vi "PidLowFirstHmi.vi"() -> ()   [LabVIEW 2018, in "Pid.lvlib"]
uses:
  Pid.lvlib
  <vilib>/Platform/TimedLoop/XDataNode/timing_clust.ctl
  <vilib>/Platform/TimedLoop/XDataNode/nitl_modes.ctl
  <vilib>/Platform/TimedLoop/XDataNode/wakeup.ctl
  <vilib>/platform/TimedLoop/XDataNode/XDataNode.xnode
  <vilib>/Platform/TimedLoop/XDataNode/XDNodeRunTimeDep.lvlib
panel:
  in  "Tune with T":bool
  in  "Update now":bool
  in  "Update rate":dbl(slide) scale=0.0..10.0
  out "Loop and out":errorcluster
  out "Modbus":errorcluster
  out "File":errorcluster
  in  "Scale":bool
  in  "Apply Max time":bool
  in  "Max time":dbl
  in  "Start/stop file":bool
  in  "Td":bool
  in  "Ti":bool
  in  "Kd":bool
  in  "Ki":bool
  in  "Kp":bool
  in  "Set Td":sgl
  in  "Set Ti":sgl
  in  "Set Ki":sgl
  in  "Set Kp":sgl
  in  "Set Kd":sgl
  out "Current Td":sgl
  out "Current Ti":sgl
  out "Current Kd":sgl
  out "Current Ki":sgl
  out "Current Kp":sgl
  out "Single Update (Multiple Plots, stacked)":cluster{"Temperature":sgl, "Setpoint":sgl, sgl}(graph)
  out "Time (ms)":u32
  out "Logging to file":bool
  in  "disable buffering (F)":bool
  out "Canceled":bool
  in  "Delimiter":string(combo)
  in  "Format":string(combo)
  out "Communication Failure":bool
  out "Off Hook":bool
  out "Updating":bool
  in  "Frequency":dbl(slide) scale=1.0..100.0
  in  "Stop":bool
  out "Counter":i32
  out "Interval":i64
  in  "file path (use dialog)":path
  in  "Setpoint":bool
  in  "Setpoint":sgl(slide) scale=0.0..255.0
  in  "Manual":bool
  in  "Manual":i16(slide) scale=0.0..255.0
  out "Setpoint":sgl(knob) scale=0.0..300.0
  out "Manual":i16(knob) scale=0.0..255.0
  out "Output":i16(knob) scale=0.0..255.0
  out "Temperature":sgl(slide) scale=0.0..300.0
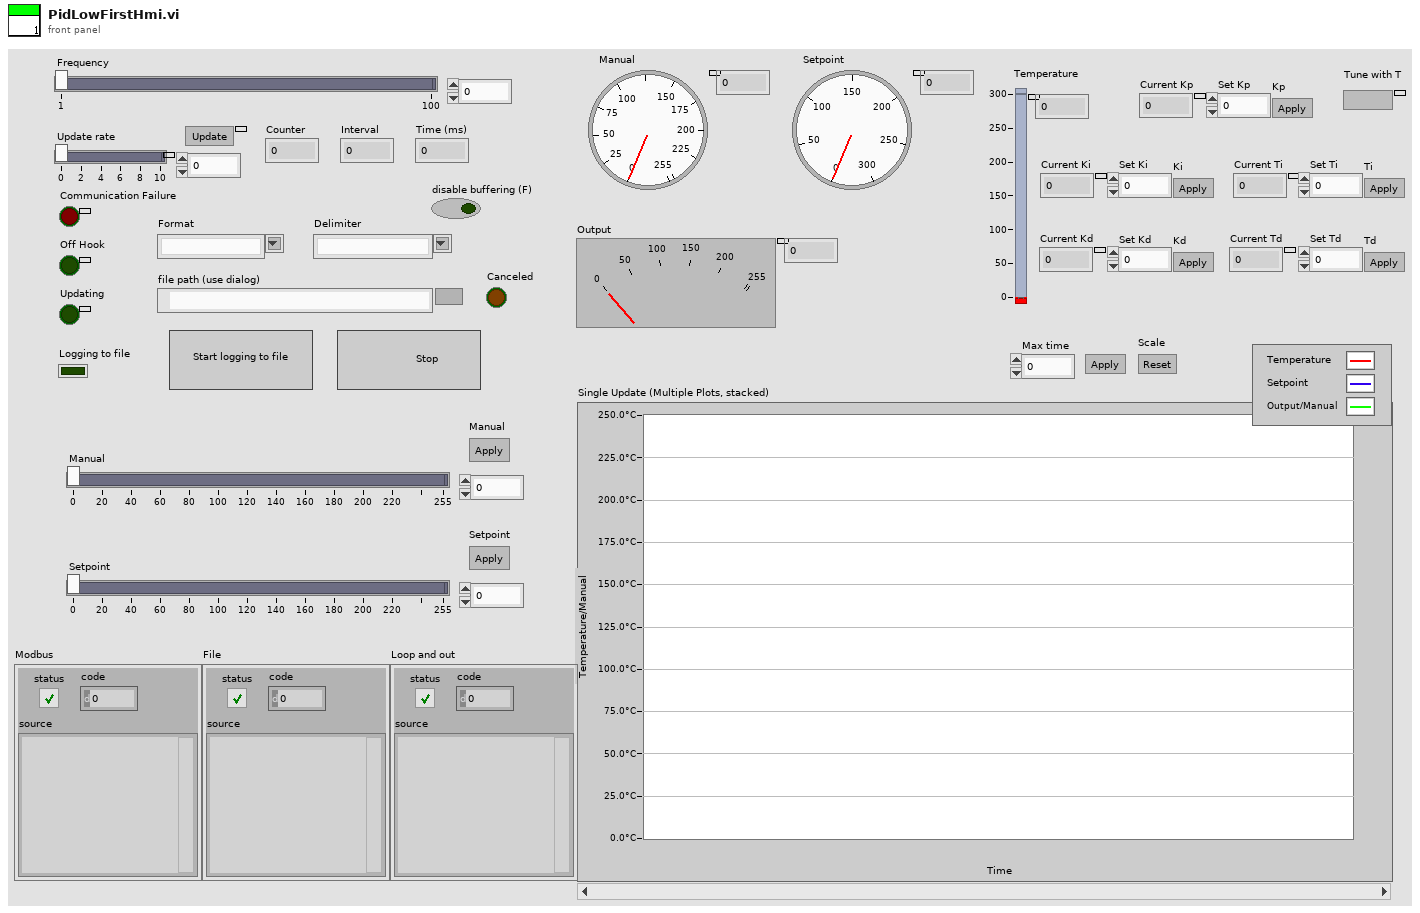
[diagram p1: front panel]
types:
  T1 = enum16{"open", "replace", "create", "open or create", "replace or create", "replace or create with confirmation"}
  T2 = typedef "XDNodeRunTimeDep.lvlib/timing_clust.ctl" = cluster{"Expected End [f-1]":u64, "Actual End [f-1]":u64, "Finished Late? [f-1]":bool, "Expected End [i-1]":u64, "Actual End [i-1]":u64, "Finished Late? [i-1]":bool, "Expected Start [i]":u64, "Actual Start [i]":u64, "Expected Start [f]":u64, "Actual Start [f]":u64, "Source Name":string, "Structure Name":string, "Period":i64, "Deadline":i64, "Offset":i64, "Start":i64, "Priority":i32, "Timeout":i32, "Mode":T3, "Wakeup Reason":T4, "Error":errorcluster, "Source Type":string, "Secondary Source Type":string, "Global End Time":u64, "Global Start Time":u64, "Frame Duration":u64, "Iteration Duration":u64, "Assigned CPU":i32, "I/O Scan Engine Mode":u32}
  T3 = typedef "XDNodeRunTimeDep.lvlib/nitl_modes.ctl" = enum32{"No Change", "Process missed periods, maintain original phase", "Discard missed periods, maintain original phase", "Process missed periods, ignore original phase", "Discard missed periods, ignore original phase"}
  T4 = typedef "XDNodeRunTimeDep.lvlib/wakeup.ctl" = enum32{"Normal", "Aborted", "Asynchronous wakeup", "Timing source error", "Timed loop error", "Timeout"}
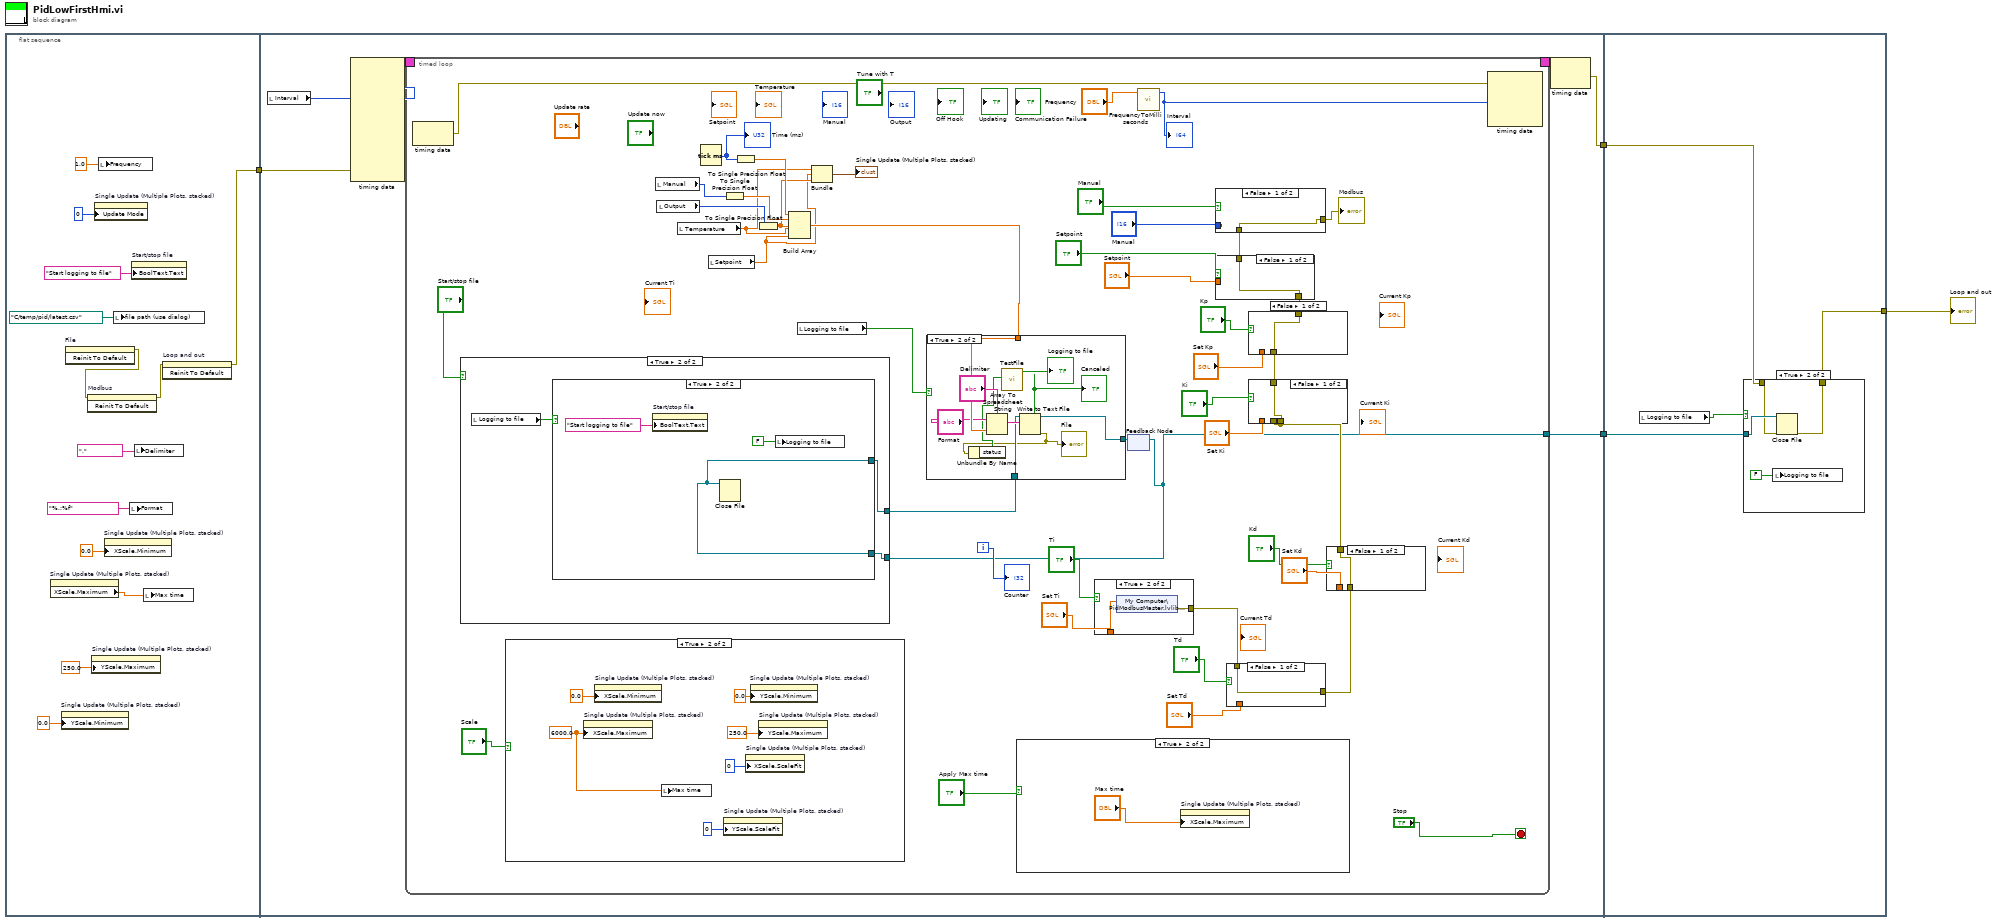
[diagram p0: block diagram]
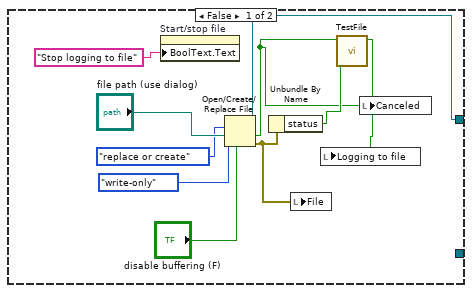
[diagram p5: hidden frame]
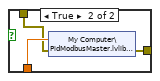
[diagram p6: hidden frame]
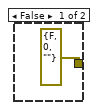
[diagram p7: hidden frame]
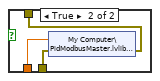
[diagram p8: hidden frame]
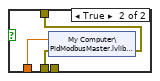
[diagram p9: hidden frame]
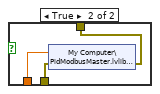
[diagram p10: hidden frame]
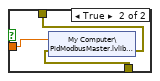
[diagram p11: hidden frame]
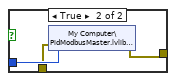
[diagram p13: hidden frame]
diagram:
  n1 = flat-sequence {
    tunnel: [w7] -> w1
    tunnel: [w20] -> w4
    tunnel: [w19] -> w3
    tunnel: w1 -> [w18]
    tunnel: w4 -> [w142]
    tunnel: w3 -> [w143]
    tunnel: [w141] -> w2
    frame #0 {
      n2 = property on="Single Update (Multiple Plots, stacked)" class="WFChart (strict)"() -> ("XScale.Maximum"=w13:dbl)  [unwired: 2 in, 2 out]
      n3 = property on="Single Update (Multiple Plots, stacked)" class="WFChart (strict)"("YScale.Minimum"=0.0 ("Y Scale.Range:Minimum")) -> ()  [unwired: 2 in, 2 out]
      n4 = invoke on="File" class="Clust (strict)" method="Reinit To Default"() -> (error out=w9:errorcluster)  [unwired: 3 in, 2 out]
      n5 = invoke on="Modbus" class="Clust (strict)" method="Reinit To Default"(error in=w9) -> (error out=w8:errorcluster)  [unwired: 2 in, 2 out]
      n6 = property on="Single Update (Multiple Plots, stacked)" class="WFChart (strict)"("YScale.Maximum"=250.0 ("Y Scale.Range:Maximum")) -> ()  [unwired: 2 in, 2 out]
      n7 = property on="Single Update (Multiple Plots, stacked)" class="WFChart (strict)"("Update Mode"=u8 0) -> ()  [unwired: 2 in, 2 out]
      n8 = local write "Frequency"(1.0 ("Frequency")) -> ()
      n9 = property on="Single Update (Multiple Plots, stacked)" class="WFChart (strict)"("XScale.Minimum"=0.0 ("X Scale.Range:Minimum")) -> ()  [unwired: 2 in, 2 out]
      n10 = local write "file path (use dialog)"(path "C:/temp/pid/latest.csv" ("file path (use dialog)")) -> ()
      n11 = local write "Format"("%.;%f" ("Format")) -> ()
      n12 = property on="Start/stop file" class="Bool"("BoolText.Text"="Start logging to file" ("Boolean Text.Text")) -> ()  [unwired: 2 in, 2 out]
      n13 = local write "Delimiter"("," ("Delimiter")) -> ()
      n14 = local write "Max time"(w13) -> ()
      n15 = invoke on="Loop and out" class="Clust (strict)" method="Reinit To Default"(error in=w8) -> (error out=w7:errorcluster)  [unwired: 2 in, 2 out]
    }
    frame #1 {
      n16 = local read "Interval"() -> (w21:i64)
      n17 = node-c288(w21, w18) -> (w23:T2)  [unwired: 8 in]
      n18 = timed-loop {
        timing: w23 -> [_]
        timing-out: [_] -> w22
        tunnel: [w35] -> w19
        i -> [w64]
        stop <- "Stop" stop-if-true
        n19 = node-c288() -> (w26:errorcluster)  [unwired: 1 in]
        n20 = case shown="True" "Scale" {
          frame False {
          }
          frame True {
            w70 = 6000.0 ("X Scale.Range:Maximum")
            n21 = property on="Single Update (Multiple Plots, stacked)" class="WFChart (strict)"("XScale.Maximum"=w70) -> ()  [unwired: 2 in, 2 out]
            n22 = property on="Single Update (Multiple Plots, stacked)" class="WFChart (strict)"("XScale.Minimum"=0.0 ("X Scale.Range:Minimum")) -> ()  [unwired: 2 in, 2 out]
            n23 = local write "Max time"(w70) -> ()
            n24 = property on="Single Update (Multiple Plots, stacked)" class="WFChart (strict)"("YScale.ScaleFit"=u8 0 ("Y Scale.Scale Fit")) -> ()  [unwired: 2 in, 2 out]
            n25 = property on="Single Update (Multiple Plots, stacked)" class="WFChart (strict)"("XScale.ScaleFit"=u8 0 ("X Scale.Scale Fit")) -> ()  [unwired: 2 in, 2 out]
            n26 = property on="Single Update (Multiple Plots, stacked)" class="WFChart (strict)"("YScale.Minimum"=0.0 ("Y Scale.Range:Minimum")) -> ()  [unwired: 2 in, 2 out]
            n27 = property on="Single Update (Multiple Plots, stacked)" class="WFChart (strict)"("YScale.Maximum"=250.0 ("Y Scale.Range:Maximum")) -> ()  [unwired: 2 in, 2 out]
          }
        }
        n28 = local read "Manual"() -> (w39:i16)
        n29 = local read "Output"() -> (w40:i16)
        n30 = local read "Temperature"() -> (w33:sgl)
        n31 = Tick Count (ms)() -> (millisecond timer value=w59:u32)
        "Time (ms)" <- w59
        n32 = local read "Setpoint"() -> (w31:sgl)
        n33 = To Single Precision Float(number=w39) -> (single precision float=w58:sgl)
        n34 = To Single Precision Float(number=w59) -> (single precision float=w60:sgl)
        n35 = To Single Precision Float(number=w40) -> (single precision float=w32:sgl)
        n36 = Build Array(w60, w58, w32, w33, w31) -> (w61:sgl[])
        n37 = local read "Logging to file"() -> (w34:bool)
        n38 = Bundle("Temperature"=w33, "Setpoint"=w31, w32) -> (→"Single Update (Multiple Plots, stacked)":cluster{"Temperature":sgl, "Setpoint":sgl, sgl})  [unwired: 1 in]
        n39 = case shown="True" "Apply Max time" {
          frame False {
          }
          frame True {
            n40 = property on="Single Update (Multiple Plots, stacked)" class="WFChart (strict)"("XScale.Maximum"="Max time") -> ()  [unwired: 2 in, 2 out]
          }
        }
        n41 = case shown="True" "Ti" {
          tunnel: "Set Ti" -> [_ w97]
          tunnel: [errorcluster {"status"=FALSE, "code"=0, "source"=""} ("error IO") w96] -> w25
          frame False {
          }
          frame True {
            n42 = shared-variable "My Computer\\PidModbusMaster.lvlib\\F400010"(w97) -> (error out=w96:errorcluster)  [unwired: 1 in]
          }
        }
        n43 = feedback #1() -> (w35:refnum<file>)  [unwired: 1 in]
        n44 = case shown="True" "Start/stop file" {
          tunnel: [w74 w76] -> w38
          tunnel: w35 -> [w74 w75]
          frame False {
          }
          frame True {
            n45 = local read "Logging to file"() -> (w77:bool)
            n46 = case shown="True" w77 {
              tunnel: [w81 w89] -> w76
              tunnel: w75 -> [_ w89]
              frame False {
                n47 = property on="Start/stop file" class="Bool"("BoolText.Text"="Stop logging to file" ("Boolean Text.Text")) -> ()  [unwired: 2 in, 2 out]
                n48 = Open/Create/Replace File(file path (use dialog)="file path (use dialog)", operation (0:open)=T1."replace or create", access (0:read/write)=enum16{"read/write", "read-only", "write-only"}."write-only", disable buffering (F)="disable buffering (F)") -> (refnum out=w81:refnum<file>, cancelled=w82:bool, error out=w78:errorcluster)  [unwired: 2 in]
                n49 = Unbundle By Name(w78) -> ("status"=w83:bool)
                n50 = local write "File"(w78) -> ()
                n51 = call "TestFile.vi"("status"=w83, "cancelled"=w82) -> ("IsOpen"=w84:bool)  [unwired: 9 in]
                n52 = local write "Logging to file"(w84) -> ()
                n53 = local write "Canceled"(w82) -> ()
              }
              frame True {
                n54 = property on="Start/stop file" class="Bool"("BoolText.Text"="Start logging to file" ("Boolean Text.Text")) -> ()  [unwired: 2 in, 2 out]
                n55 = Close File(refnum=w89) -> ()  [unwired: 1 in, 2 out]
                n56 = local write "Logging to file"(FALSE ("Logging to file")) -> ()
              }
            }
          }
        }
        n57 = case shown="True" w34 {
          tunnel: w61 -> [_ w124]
          tunnel: [w114 w121] -> w36
          tunnel: w38 -> [w114 w119]
          frame False {
          }
          frame True {
            n58 = Array To Spreadsheet String(delimiter (Tab)="Delimiter", array=w124, 3:"Format") -> (spreadsheet string=w120:string)
            n59 = Write to Text File(file (use dialog)=w119, text=w120) -> (refnum out=w121:refnum<file>, cancelled=w117:bool, error out=w115:errorcluster)  [unwired: 2 in]
            "Canceled" <- w117
            "File" <- w115
            n60 = Unbundle By Name(w115) -> ("status"=w116:bool)
            n61 = call "TestFile.vi"("status"=w116, "cancelled"=w117) -> ("IsOpen"=→"Logging to file":bool)  [unwired: 9 in]
          }
        }
        n62 = feedback-in #1(w36) -> ()
        n63 = call "FrequencyToMilliseconds.vi"("Frequency"="Frequency") -> ("Numeric"=w65:i64)  [unwired: 10 in]
        "Interval" <- w65
        n64 = case shown="False" "Td" {
          tunnel: "Set Td" -> [_ w94]
          tunnel: [w91 w93] -> w45
          tunnel: w25 -> [w91 w92]
          frame False {
          }
          frame True {
            n65 = shared-variable "My Computer\\PidModbusMaster.lvlib\\F400012"(w94, error in=w92) -> (error out=w93:errorcluster)
          }
        }
        n66 = case shown="False" "Kd" {
          tunnel: "Set Kd" -> [_ w101]
          tunnel: w45 -> [w98 w100]
          tunnel: [w98 w99] -> w41
          frame False {
          }
          frame True {
            n67 = shared-variable "My Computer\\PidModbusMaster.lvlib\\F400008"(w101, error in=w100) -> (error out=w99:errorcluster)
          }
        }
        n68 = case shown="False" "Ki" {
          tunnel: "Set Ki" -> [_ w105]
          tunnel: w41 -> [_ w104]
          tunnel: [w102 w103] -> w44
          tunnel: w41 -> [w102 _]
          frame False {
          }
          frame True {
            n69 = shared-variable "My Computer\\PidModbusMaster.lvlib\\F400006"(w105, error in=w104) -> (error out=w103:errorcluster)
          }
        }
        n70 = case shown="False" "Kp" {
          tunnel: "Set Kp" -> [_ w109]
          tunnel: w44 -> [w106 w108]
          tunnel: [w106 w107] -> w43
          frame False {
          }
          frame True {
            n71 = shared-variable "My Computer\\PidModbusMaster.lvlib\\F400004"(w109, error in=w108) -> (error out=w107:errorcluster)
          }
        }
        n72 = case shown="False" "Setpoint" {
          tunnel: "Setpoint" -> [_ w113]
          tunnel: w43 -> [w110 w112]
          tunnel: [w110 w111] -> w42
          frame False {
          }
          frame True {
            n73 = shared-variable "My Computer\\PidModbusMaster.lvlib\\F400002"(w113, error in=w112) -> (error out=w111:errorcluster)
          }
        }
        n74 = case shown="False" "Manual" {
          tunnel: "Manual" -> [_ w128]
          tunnel: [w125 w127] -> w27
          tunnel: w42 -> [w125 w126]
          frame False {
          }
          frame True {
            n75 = shared-variable "My Computer\\PidModbusMaster.lvlib\\S400001"(w128, error in=w126) -> (error out=w127:errorcluster)
          }
        }
        "Modbus" <- w27
        n76 = node-c288(w26, w65) -> ()  [unwired: 2 in, 1 out]
        "Counter" <- w64
      }
      n77 = node-c288(w22) -> (w20:errorcluster)
    }
    frame #2 {
      n78 = local read "Logging to file"() -> (w144:bool)
      n79 = case shown="True" w144 {
        tunnel: w143 -> [_ w149]
        tunnel: w142 -> [w145 w148]
        tunnel: [w145 w147] -> w141
        frame False {
        }
        frame True {
          n80 = local write "Logging to file"(FALSE ("Logging to file")) -> ()
          n81 = Close File(refnum=w149, error in=w148) -> (error out=w147:errorcluster)  [unwired: 1 out]
        }
      }
    }
  }
  "Loop and out" <- w2
